vi "TestCodeTEST.vi"() -> ()   [LabVIEW 2018]
uses:
  Controls/Powermeter Actions.ctl
panel:
  in  "stop":bool
  out "Sensor Name":string
  out "Average Time":dbl
  in  "Average Time (0.0)":dbl=0.1
  out "Wavelength":dbl
  in  "Wavelength":dbl=930.0 caption="Wavelength (0.0)"
  out "Power":dbl
  out "error out":errorcluster
  in  "error in (no error)":errorcluster {"code" format="%.0x"}
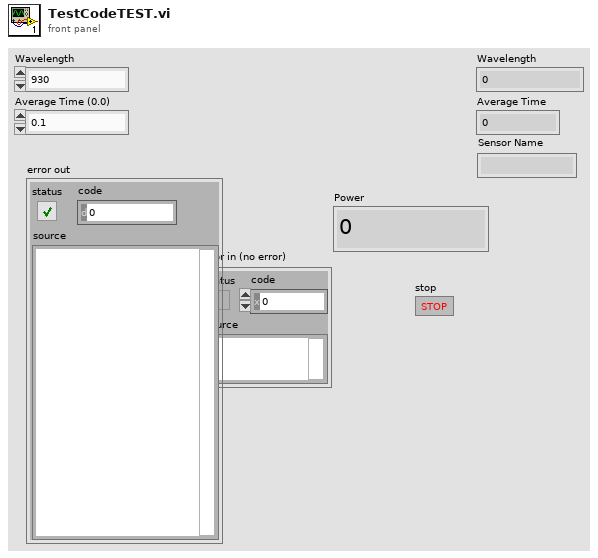
[diagram p1: front panel]
types:
  T1 = typedef "Powermeter Actions.ctl" = enum16{"Init", "Set-Get Avg", "Set-Get Wavelength", "Do measure"}
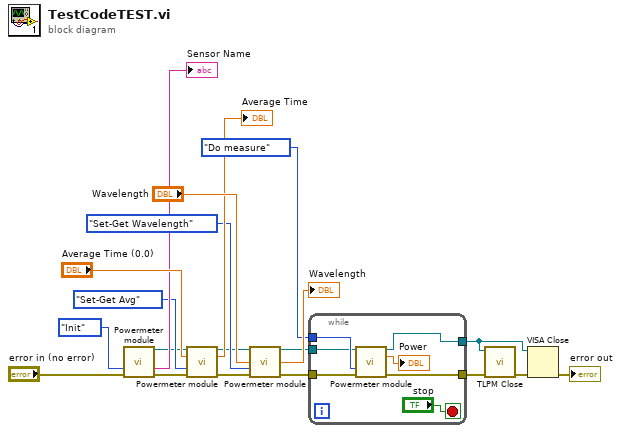
[diagram p0: block diagram]
diagram:
  n1 = call "Powermeter module.vi"("Enum"=Powermeter_Actions."Init", "error in (no error)"="error in (no error)") -> ("instrument handle 2"=w3:refnum<visa-resource-name>, "Sensor Name"=→"Sensor Name":string, "error out"=w19:errorcluster)  [unwired: 9 in, 2 out]
  n2 = call "Powermeter module.vi"("instrument handle"=w3, "Average Time (0.0)"="Average Time (0.0)", "Enum"=Powermeter_Actions."Set-Get Avg", "error in (no error)"=w19) -> ("instrument handle 2"=w2:refnum<visa-resource-name>, "Average Time"=→"Average Time":dbl, "error out"=w18:errorcluster)  [unwired: 7 in, 2 out]
  n3 = call "Powermeter module.vi"("instrument handle"=w2, "Wavelength"="Wavelength", "Enum"=Powermeter_Actions."Set-Get Wavelength", "error in (no error)"=w18) -> ("instrument handle 2"=w1:refnum<visa-resource-name>, "Wavelength"=→"Wavelength":dbl, "error out"=w17:errorcluster)  [unwired: 7 in, 2 out]
  n4 = while {
    tunnel: w17 -> [w27]
    tunnel: [w26] -> w10
    tunnel: [w23] -> w8
    tunnel: Powermeter_Actions."Do measure" -> [w22]
    tunnel: w1 -> [w21]
    stop <- "stop" stop-if-true
    n5 = call "Powermeter module.vi"("instrument handle"=w21, "Enum"=w22, "error in (no error)"=w27) -> ("instrument handle 2"=w23:refnum<visa-resource-name>, "Average Time"=→"Power":dbl, "error out"=w26:errorcluster)  [unwired: 8 in, 2 out]
  }
  n6 = call "TLPM Close.vi"("error in (no error)"=w10, "instrument handle"=w8) -> ("error out"=w11:errorcluster)  [unwired: 9 in]
  n7 = VISA Close(VISA resource name=w8, error in (no error)=w11) -> (error out=→"error out":errorcluster)
